vi "Simple Auto-Shifter.vi"(0 "x":dbl=60.0, 2 "y":dbl=60.0, 3 "Manual Power Override":bool=TRUE, 5 "Manual Speed Override":bool=TRUE, 9 "Shift Solenoid":T1={"DevStatus"={"status"=FALSE, "code"=0, "source"=""}, "Solenoid Module"=enum."Solenoid Module 1", "Forward Solenoid Channel"=enum."Invalid", "Reverse Solenoid Channel"=enum."Invalid"}, 10 "Left Enc":T4={"DevStatus"={"status"=FALSE, "code"=0, "source"=""}, "EncoderIndex"=enum."Enc 0", "CounterIndex"=enum."Ctr 0", "DistancePerCount"=1.0, "Decoding Type"=enum."4x"}) -> (19 "Speed Gear?":bool)   [LabVIEW 2012]
uses:
  <vilib>/Rock Robotics/WPI/Encoder/WPI_EncoderDevRef.ctl
  <vilib>/Rock Robotics/SystemInterfaces/Encoder/FPGA_EncoderIdx.ctl
  <vilib>/Rock Robotics/SystemInterfaces/Counter/FPGA_CounterCtrSystemIndex.ctl
  <vilib>/Rock Robotics/WPI/Encoder/WPI_EncoderType.ctl
  <vilib>/Rock Robotics/WPI/Solenoid/WPI_SolenoidDevRef.ctl
  <vilib>/Rock Robotics/SystemInterfaces/Typedef/FPGA_TypedefSolenoidModule.ctl
  <vilib>/Rock Robotics/WPI/Solenoid/WPI_SolenoidChannel.ctl
  <vilib>/Rock Robotics/WPI/Solenoid/WPI_SolenoidValue.ctl
  <vilib>/Rock Robotics/WPI/Solenoid/WPI_SolenoidSetEnum.vi
panel:
  out "Waveform Chart":cluster{dbl, i16}(graph)
  in  "Delta":dbl
  in  "Limit":dbl
  out "Distance":dbl
  in  "Low Limit":dbl=0.8
  in  "High Limit":dbl=1.2
  out "RPM":dbl
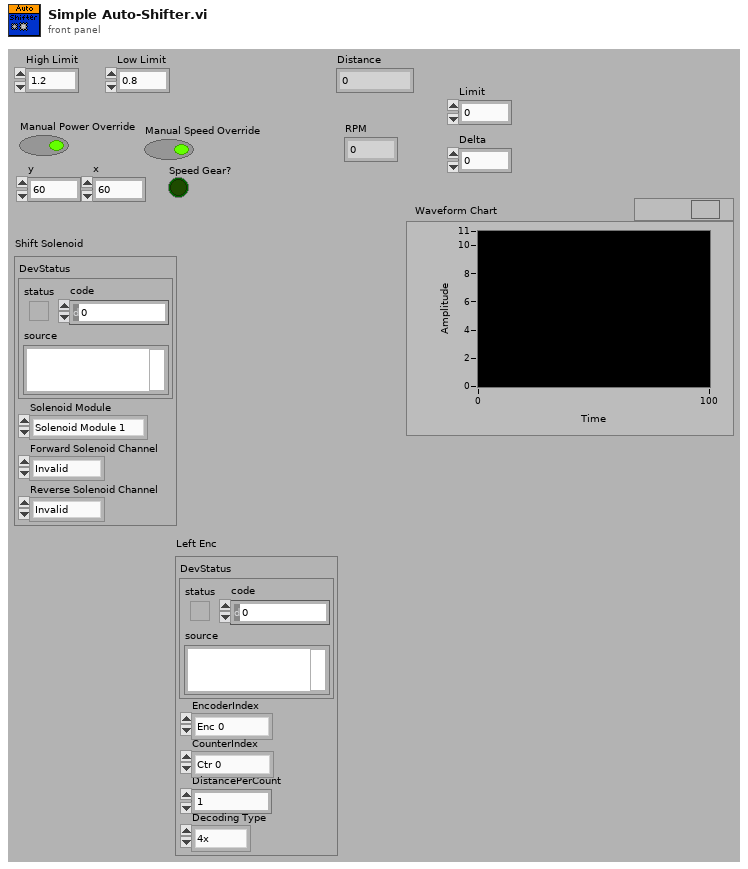
[diagram p1: front panel]
types:
  T1 = typedef "WPI_SolenoidDevRef.ctl" = cluster{"DevStatus":errorcluster, "Solenoid Module":T2, "Forward Solenoid Channel":T3, "Reverse Solenoid Channel":T3}
  T2 = typedef "FPGA_TypedefSolenoidModule.ctl" = enum16{"Solenoid Module 1", "Solenoid Module 2"}
  T3 = typedef "WPI_SolenoidChannel.ctl" = enum8{"Solenoid 1", "Solenoid 2", "Solenoid 3", "Solenoid 4", "Solenoid 5", "Solenoid 6", "Solenoid 7", "Solenoid 8", "Invalid"}
  T4 = typedef "WPI_EncoderDevRef.ctl" = cluster{"DevStatus":errorcluster, "EncoderIndex":T5, "CounterIndex":T6, "DistancePerCount":dbl, "Decoding Type":T7}
  T5 = typedef "FPGA_EncoderIdx.ctl" = enum8{"Enc 0", "Enc 1", "Enc 2", "Enc 3", "Invalid"}
  T6 = typedef "FPGA_CounterCtrSystemIndex.ctl" = enum8{"Ctr 0", "Ctr 1", "Ctr 2", "Ctr 3", "Ctr 4", "Ctr 5", "Ctr 6", "Ctr 7", "Invalid"}
  T7 = typedef "WPI_EncoderType.ctl" = enum16{"1x", "2x", "4x"}
  T8 = typedef "WPI_SolenoidValue.ctl" = enum16{"Off", "On", "Forward", "Reverse"}
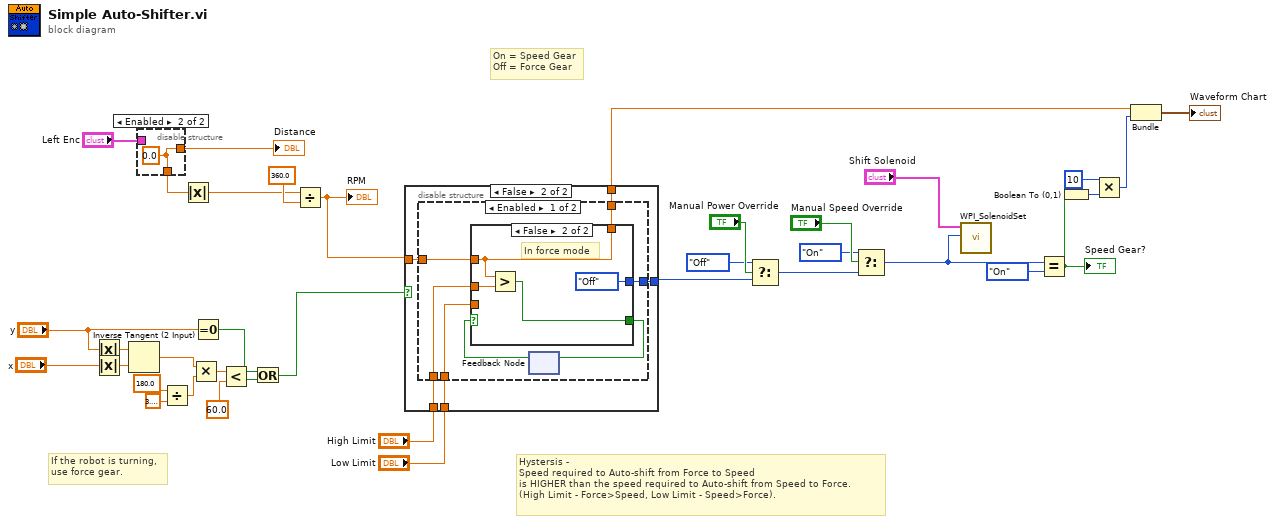
[diagram p0: block diagram]
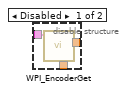
[diagram p2: hidden frame]
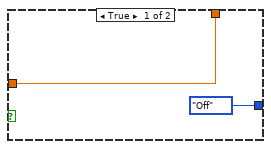
[diagram p3: hidden frame]
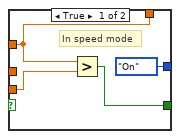
[diagram p4: hidden frame]
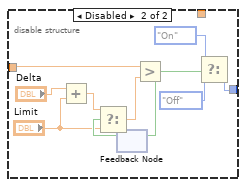
[diagram p5: hidden frame]
diagram:
  # "Hystersis - \nSpeed required to Auto-shift from Force to Speed\nis HIGHER than the speed required to Auto-shift from Speed to Force.\n(High Limit - Force>Speed, Low Limit - Speed>Force)."
  # "On = Speed Gear\nOff = Force Gear"
  # "If the robot is turning,\nuse force gear."
  n1 = Absolute Value(x="y") -> (abs(x)=w8:dbl)
  n2 = Absolute Value(x="x") -> (abs(x)=w7:dbl)
  n3 = Inverse Tangent (2 Input)(1:w7, 2:w8) -> (0:w4:dbl)
  n4 = disable-structure shown="Enabled" {
    disable-tunnel: "Left Enc" -> [w39 _]
    disable-tunnel: [w38 w40] -> w23
    disable-tunnel: [w37 w40] -> w15
    frame Disabled {
      n5 = call <vilib>:"WPI_EncoderGet.vi"("EncoderDevRef"=w39) -> ("Distance"=w38:dbl, "Rate"=w37:dbl)  [unwired: 1 in, 8 out]
    }
    frame Enabled {
      w40 = 0.0 ("y")
    }
  }
  "Distance" <- w23
  n6 = Divide(x=180.0 ("atan2(y,x)"), y=3.141592653589793) -> (x/y=w3:dbl)
  n7 = Absolute Value(x=w15) -> (abs(x)=w14:dbl)
  n8 = Multiply(x=w4, y=w3) -> (x*y=w5:dbl)
  n9 = Equal To 0?(x="y") -> (x = 0?=w10:bool)
  n10 = Less?(x=w5, y=60.0 ("atan2(y,x)")) -> (x < y?=w9:bool)
  n11 = Or(x=w10, y=w9) -> (x .or. y?=w11:bool)
  n12 = Divide(x=w14, y=360.0) -> (x/y=w31:dbl)
  "RPM" <- w31
  n13 = case shown="False" w11 {
    tunnel: [WPI_SolenoidValue."Off" ("Value") w47] -> w32
    tunnel: w31 -> [w41 w46]
    tunnel: "High Limit" -> [_ w45]
    tunnel: "Low Limit" -> [_ w44]
    tunnel: [w41 w43] -> w16
    frame True {
    }
    frame False {
      n14 = disable-structure shown="Enabled" {
        disable-tunnel: [w52 w71] -> w47
        disable-tunnel: w46 -> [w51 w72]
        disable-tunnel: w45 -> [w50 _]
        disable-tunnel: w44 -> [w49 _]
        disable-tunnel: [w48 _] -> w43
        frame Enabled {
          n15 = feedback #1() -> (w53:bool)  [unwired: 1 out]
          n16 = case shown="False" w53 {
            tunnel: w51 -> [w55 w59]
            tunnel: [w58 w62] -> w54
            tunnel: [WPI_SolenoidValue."On" ("Value") WPI_SolenoidValue."Off" ("Value")] -> w52
            tunnel: w50 -> [_ w60]
            tunnel: w49 -> [w56 _]
            tunnel: [w55 w59] -> w48
            frame True {
              # "In speed mode"
              n17 = Greater?(x=w55, y=w56) -> (0:w58:bool)
            }
            frame False {
              # "In force mode"
              n18 = Greater?(x=w59, y=w60) -> (0:w62:bool)
            }
          }
          n19 = feedback-in #1(w54) -> ()
        }
        frame Disabled {
          n20 = Add(x="Delta", y="Limit") -> (x+y=w65:dbl)
          n21 = feedback #2() -> (w66:bool)  [unwired: 1 out]
          n22 = Select(t=w65, s=w66, f="Limit") -> (s? t:f=w68:dbl)
          n23 = Greater?(x=w72, y=w68) -> (0:w67:bool)
          n24 = feedback-in #2(w67) -> ()
          n25 = Select(t=WPI_SolenoidValue."On" ("Value"), s=w67, f=WPI_SolenoidValue."Off" ("Value")) -> (s? t:f=w71:T8)
        }
      }
    }
  }
  n26 = Select(t=WPI_SolenoidValue."Off" ("Value"), s="Manual Power Override", f=w32) -> (s? t:f=w27:T8)
  n27 = Select(t=WPI_SolenoidValue."On", s="Manual Speed Override", f=w27) -> (s? t:f=w21:T8)
  n28 = call-poly <vilib>:"WPI_SolenoidSet.vi"("Value"=w21, "SolenoidDevRef"="Shift Solenoid") -> ()  [unwired: 1 in, 9 out]
  n29 = Equal?(x=w21, y=WPI_SolenoidValue."On") -> (x = y?=w20:bool)
  "Speed Gear?" <- w20
  n30 = Boolean To (0,1)(Boolean=w20) -> (0, 1=w19:i16)
  n31 = Multiply(x=i16 10, y=w19) -> (x*y=w17:i16)
  n32 = Bundle(w16, w17) -> (→"Waveform Chart":cluster{dbl, i16})  [unwired: 1 out]
